vi "M01 Wind Turbine.vi"   [LabVIEW 2016]
uses:
  <vilib>/NXT/Block Support/NXT_InputPort.ctl
  <vilib>/NXT/Block Support/NXT_OutputPort.ctl
  <vilib>/NXT/NXTIO Xnodes/NXTIONodeSubVIs/NXTMotorRunDistance.vi
  <vilib>/NXT/NXTIO Xnodes/AddressXNode/NXTIOAddress.xnode
  <vilib>/NXT/NXTIO Xnodes/NXTIOXNode/NXTIO.xnode
  <vilib>/NXT/Subs/LVHSConnector.ctl
  <vilib>/NXT/LegoClasses/BrickReference/BrickReference.lvclass
types:
  T1 = typedef "NXT_OutputPort.ctl" = u8
  T2 = typedef "NXT_InputPort.ctl" = u32
  T3 = typedef "LVHSConnector.ctl" = refnum<class "BrickReference.lvclass">
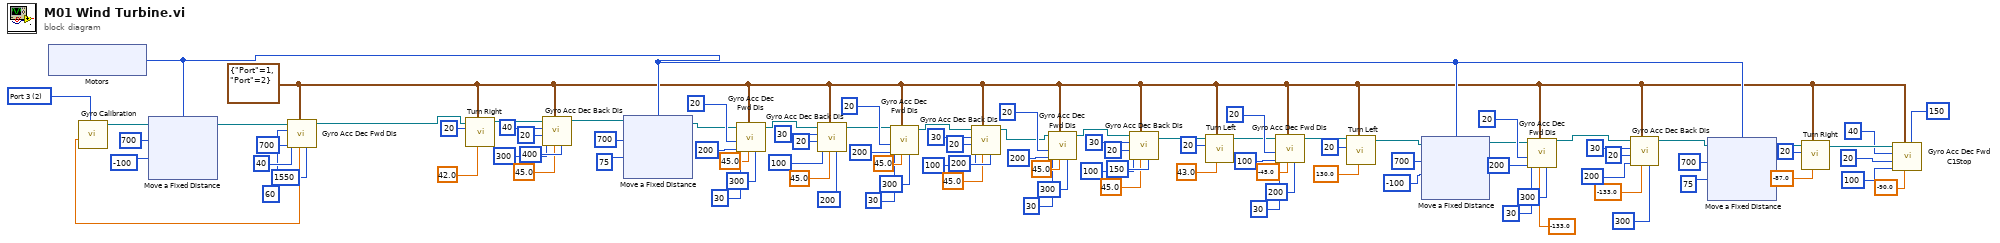
[diagram p0: block diagram]
diagram:
  w6 = cluster{"Port":T1, "Port":T1} {"Port"=1, "Port"=2} ("Motor")
  w99 = T2 2 items=["Port 1", "Port 2", "Port 3", "Port 4"] ("Port (Port 1)")
  n1 = xnode "Motors"() -> ("Motor"=w11:T1)
  n2 = call "Gyro Calibration.vi"("Port (Port 1)"=w99) -> ("Degrees"=w95:sgl, "NXT/EV3"=w98:T3)  [unwired: 6 in, 1 out]
  n3 = xnode "Move a Fixed Distance"("Speed 1"=i8 -100, "Distance 1"=700, "Motors"=w11, "NXT/EV3"=w98) -> ("NXT/EV3"=w21:T3)
  n4 = call "Gyro Acc Dec Fwd Dis.vi"("Stop rotation"=1550, "Ini. Degrees"=w95, "Motor"=w6, "Threshold to De-acc"=700, "De-acc"=40, "Acc"=60, "EV3 in"=w21) -> ("EV3 out"=w22:T3)  [unwired: 4 in]
  n5 = call "Turn Right.vi"("Turning angle"=sgl 42.0, "Motor"=w6, "Motor B (right)"=i8 20, "EV3 in"=w22) -> ("EV3 out"=w88:T3)  [unwired: 7 in]
  n6 = call "Gyro Acc Dec Back Dis.vi"("Stop rotation"=400, "Ini. Degrees"=sgl 45.0, "Motor"=w6, "Threshold to De-acc"=300, "De-acc"=20, "Acc"=40, "EV3 in"=w88) -> ("EV3 out"=w80:T3)  [unwired: 4 in]
  n7 = xnode "Move a Fixed Distance"("Speed 1"=i8 75, "Distance 1"=700, "Motors"=w11, "NXT/EV3"=w80) -> ("NXT/EV3"=w75:T3)
  n8 = call "Gyro Acc Dec Fwd Dis.vi"("Stop rotation"=300, "Ini. Degrees"=sgl 45.0, "Motor"=w6, "Threshold to De-acc"=200, "De-acc"=20, "Acc"=30, "EV3 in"=w75) -> ("EV3 out"=w68:T3)  [unwired: 4 in]
  n9 = call "Gyro Acc Dec Back Dis.vi"("Stop rotation"=200, "Ini. Degrees"=sgl 45.0, "Motor"=w6, "Threshold to De-acc"=100, "De-acc"=20, "Acc"=30, "EV3 in"=w68) -> ("EV3 out"=w56:T3)  [unwired: 4 in]
  n10 = call "Gyro Acc Dec Fwd Dis.vi"("Stop rotation"=300, "Ini. Degrees"=sgl 45.0, "Motor"=w6, "Threshold to De-acc"=200, "De-acc"=20, "Acc"=30, "EV3 in"=w56) -> ("EV3 out"=w67:T3)  [unwired: 4 in]
  n11 = call "Gyro Acc Dec Back Dis.vi"("Stop rotation"=200, "Ini. Degrees"=sgl 45.0, "Motor"=w6, "Threshold to De-acc"=100, "De-acc"=20, "Acc"=30, "EV3 in"=w67) -> ("EV3 out"=w44:T3)  [unwired: 4 in]
  n12 = call "Gyro Acc Dec Fwd Dis.vi"("Stop rotation"=300, "Ini. Degrees"=sgl 45.0, "Motor"=w6, "Threshold to De-acc"=200, "De-acc"=20, "Acc"=30, "EV3 in"=w44) -> ("EV3 out"=w55:T3)  [unwired: 4 in]
  n13 = call "Gyro Acc Dec Back Dis.vi"("Stop rotation"=150, "Ini. Degrees"=sgl 45.0, "Motor"=w6, "Threshold to De-acc"=100, "De-acc"=20, "Acc"=30, "EV3 in"=w55) -> ("EV3 out"=w43:T3)  [unwired: 4 in]
  n14 = call "Turn Left.vi"("Turning angle"=sgl 43.0, "Motor"=w6, "Motor B (right)"=i8 20, "EV3 in"=w43) -> ("EV3 out"=w36:T3)  [unwired: 7 in]
  n15 = call "Gyro Acc Dec Fwd Dis.vi"("Stop rotation"=200, "Ini. Degrees"=sgl -45.0, "Motor"=w6, "Threshold to De-acc"=100, "De-acc"=20, "Acc"=30, "EV3 in"=w36) -> ("EV3 out"=w34:T3)  [unwired: 4 in]
  n16 = call "Turn Left.vi"("Turning angle"=sgl 130.0, "Motor"=w6, "Motor B (right)"=i8 20, "EV3 in"=w34) -> ("EV3 out"=w30:T3)  [unwired: 7 in]
  n17 = xnode "Move a Fixed Distance"("Speed 1"=i8 -100, "Distance 1"=700, "Motors"=w11, "NXT/EV3"=w30) -> ("NXT/EV3"=w23:T3)
  n18 = call "Gyro Acc Dec Fwd Dis.vi"("Stop rotation"=300, "Ini. Degrees"=sgl -133.0, "Motor"=w6, "Threshold to De-acc"=200, "De-acc"=20, "Acc"=30, "EV3 in"=w23) -> ("EV3 out"=w15:T3)  [unwired: 4 in]
  n19 = call "Gyro Acc Dec Back Dis.vi"("Stop rotation"=300, "Ini. Degrees"=sgl -133.0, "Motor"=w6, "Threshold to De-acc"=200, "De-acc"=20, "Acc"=30, "EV3 in"=w15) -> ("EV3 out"=w12:T3)  [unwired: 4 in]
  n20 = xnode "Move a Fixed Distance"("Speed 1"=i8 75, "Distance 1"=700, "Motors"=w11, "NXT/EV3"=w12) -> ("NXT/EV3"=w10:T3)
  n21 = call "Turn Right.vi"("Turning angle"=sgl -87.0, "Motor"=w6, "Motor B (right)"=i8 20, "EV3 in"=w10) -> ("EV3 out"=w7:T3)  [unwired: 7 in]
  n22 = call "Gyro Acc Dec Fwd C1Stop.vi"("Threshold to C1"=150, "Ini. Degrees"=sgl -90.0, "Motor"=w6, "Threshold to De-acc"=100, "De-acc"=20, "Acc"=40, "EV3 in"=w7) -> ()  [unwired: 4 in, 1 out]
